vi "PS90_MotorInit.vi"(3 "error in (no error)":errorcluster, 4 "Axis number":i32=1 min=1 max=9, 5 "Control unit ID":i32=1 min=1 max=10, 6 "DLOwis.lvclass":refnum<class "DLOwis.lvclass">) -> (0 "error out":errorcluster, 2 "DLOwis.lvclass":refnum<class "DLOwis.lvclass">)   [LabVIEW 2019, in "DLOwis.lvclass"]
doc: "PS90_MotorInit.vi, created: 17.10.2006 alex; last change: 19.07.2016 alex;\n\n<B>FUNCTION:</B> \n\nInitialize an axis and switch on.\nWith this function the axis is completely initialized and afterwards is \nwith a current and with active positioning regulator.\nIt must be executed after the turning on of the control unit, so that the\naxis can be moved afterwards with the commands REF, PGO, VGO etc.\nBefore the following parameters must have been set: limit switch mask\nand polarity, start regulator parameters.\n----------------------------------------------------------------------------------------\n<B>INPUT:</B>\n[I32] <B>Control unit ID:</B> control unit index. (Default=1, Range=1...10) \n[I32] <B>Axis number:</B> axis number. (Default=1, Range=1...9) \n[CLU] <B>error in</B>\n----------------------------------------------------------------------------------------\n<B>OUTPUT:</B>\n[CLU] <B>error out</B>\n----------------------------------------------------------------------------------------\n<B>SUB-VIs:</B>\n----------------------------------------------------------------------------------------\n<B>EXT-Calls:</B>\nps90.dll (V2.00)\n----------------------------------------------------------------------------------------"
uses:
  DLOwis.lvclass
  C:/Users/elysium/Documents/dev/TRANCON/Classes/Delay Line/DelayLine.lvclass
  DelayLine.lvclass/DelayLine.ctl
  DelayLine.lvclass
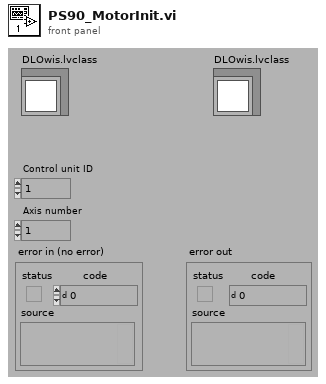
[diagram p1: front panel]
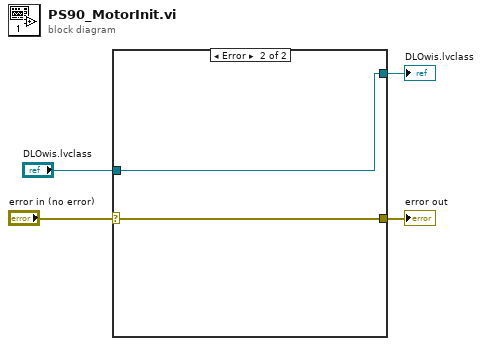
[diagram p0: block diagram]
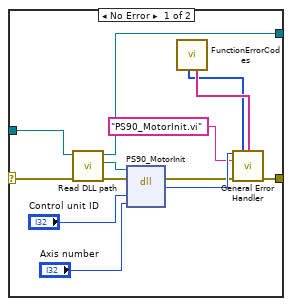
[diagram p2: hidden frame]
diagram:
  n1 = case shown="Error" "error in (no error)" {
    selector: "error in (no error)" -> [w6 w19]
    tunnel: [w16 w19] -> w4
    tunnel: "DLOwis.lvclass" -> [w7 w18]
    tunnel: [w5 w18] -> w1
    frame No Error {
      n2 = call "Read DLL path.vi"("error in (no error)"=w6, "DelayLine in"=w7) -> ("error out"=w9:errorcluster, "DLL path"=w10:path, "DelayLine out"=w5:refnum<class "DLOwis.lvclass">)  [unwired: 7 in]
      n3 = dll-call lib="C:/Users/Sergey Denisov/Documents/REPS/TRANCON/DLL/ps90.dll" fn="PS90_MotorInit"(path in=w10, error in=w9, "Index"="Control unit ID", "AxisNr"="Axis number") -> (error out=w8:errorcluster, "Rückgabetyp"=w15:i32)  [unwired: 3 in, 1 out]
      n4 = call "FunctionErrorCodes.vi"() -> ("[user-defined codes]"=w11:i32[], "[user-defined descriptions]"=w12:string[])  [unwired: 8 in]
      n5 = call <vilib>:"General Error Handler.vi"("[error code] (0)"=w15, "[user-defined codes]"=w11, "[user-defined descriptions]"=w12, "[error source] (\" \")"="PS90_MotorInit.vi" ("[error source] (\" \")"), "error in (no error)"=w8) -> ("error out"=w16:errorcluster)  [unwired: 6 in, 4 out]
    }
    frame Error {
    }
  }
  "error out" <- w4
  "DLOwis.lvclass" <- w1
